vi "Create 3D Mecanum Wheel from Params.vi"(5 "colors":T2={"wheel color"=4884736, "roller color"=590024}, 7 "dimensions":T1={"roller thickness"=0.1, "roller radius"=0.05, "frame thickness"=0.025, "number of rollers"=6, "axle radius"=0.03, "axle length"=0.5}, 8 "error in (no error)":errorcluster, 9 "roller orientation":T3 items=["Left", "Right"], 10 "wheel radius":dbl=0.25, 11 "name":string) -> (0 "error out":errorcluster, 2 "rotation axis":refnum<vi>, 3 "3D mecanum wheel frame":refnum<vi>)   [LabVIEW 2017, in "NI_Robotics 3D Picture Steering Utilities.lvlib"]
doc: "Creates a 3D picture control mecanum wheel object."
uses:
  <vilib>/robotics/Steering/Utilities/3D Picture/NI_Robotics 3D Picture Steering Utilities.lvlib
  <vilib>/robotics/Steering/Mecanum Wheel/Roller Orientation.ctl
  <vilib>/robotics/Steering/Utilities/3D Picture/Mecanum Wheel Colors.ctl
  <vilib>/robotics/Steering/Utilities/3D Picture/Mecanum Wheel Dimensions.ctl
  <vilib>/picture/3D Picture Control/Object/Create Object (name).vi
  <vilib>/picture/3D Picture Control/NI_3D Picture Control.lvlib
  <vilib>/robotics/Steering/Mecanum Wheel/NI_Robotics_Mecanum Wheel.lvclass
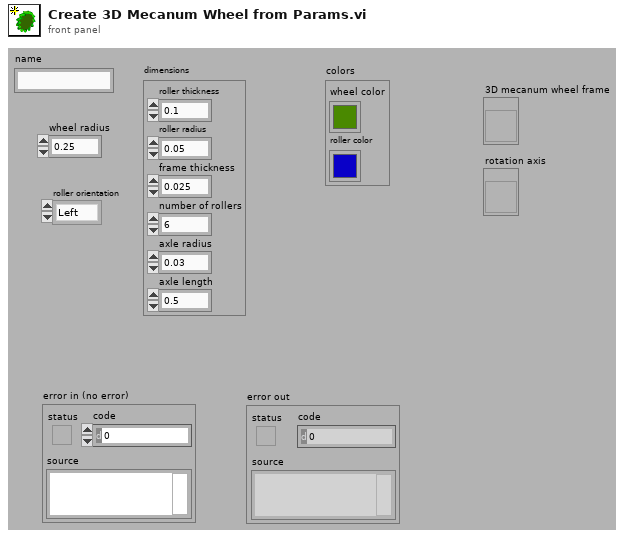
[diagram p1: front panel]
types:
  T1 = typedef "NI_Robotics 3D Picture Steering Utilities.lvlib/Mecanum Wheel Dimensions.ctl" = cluster{"roller thickness":dbl, "roller radius":dbl, "frame thickness":dbl, "number of rollers":i32, "axle radius":dbl, "axle length":dbl}
  T2 = typedef "NI_Robotics 3D Picture Steering Utilities.lvlib/Mecanum Wheel Colors.ctl" = cluster{"wheel color":u32, "roller color":u32}
  T3 = typedef "NI_Robotics_Mecanum Wheel.lvclass/Roller Orientation.ctl" = u16
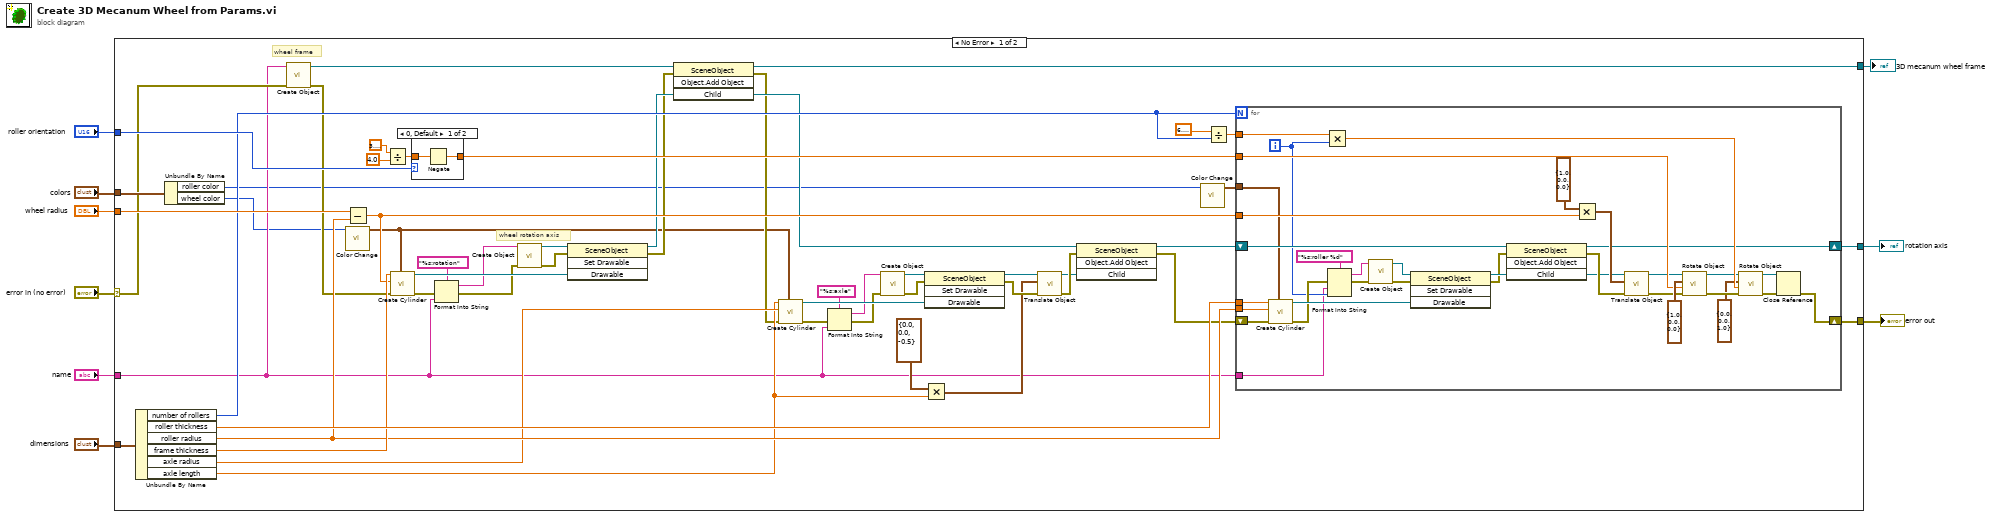
[diagram p0: block diagram]
diagram:
  n1 = case shown="No Error" "error in (no error)" {
    selector: "error in (no error)" -> [w26 w101]
    tunnel: [w59 _] -> w9
    tunnel: "dimensions" -> [w58 _]
    tunnel: "wheel radius" -> [w51 _]
    tunnel: "colors" -> [w49 _]
    tunnel: "roller orientation" -> [w28 _]
    tunnel: [w33 w101] -> w3
    tunnel: "name" -> [w15 _]
    tunnel: [w19 _] -> w1
    frame No Error {
      # "wheel rotation axis"
      # "wheel frame"
      n2 = Unbundle By Name(w58) -> ("number of rollers"=w27:i32, "roller thickness"=w57:dbl, "roller radius"=w52:dbl, "frame thickness"=w53:dbl, "axle radius"=w46:dbl, "axle length"=w36:dbl)
      n3 = Unbundle By Name(w49) -> ("roller color"=w11:u32, "wheel color"=w13:u32)
      n4 = call-poly <vilib>:"Create Object.vi"("error in (no error)"=w26, "Name"=w15) -> ("error out"=w25:errorcluster, "Scene:New Object"=w24:refnum<vi>)  [unwired: 8 in]
      n5 = call <vilib>:"Color Change.vi"("Color"=w13) -> ("RGBA"=w12:cluster{"R":sgl, "G":sgl, "B":sgl, "A":sgl})  [unwired: 10 in]
      n6 = Subtract(x=w51, y=w52) -> (x-y=w50:dbl)
      n7 = Divide(x=3.141592653589793, y=4.0) -> (x/y=w48:dbl)
      n8 = call <vilib>:"Create Cylinder.vi"("Color"=w12, "error in (no error)"=w25, "Radius"=w50, "Height"=w53) -> ("error out"=w18:errorcluster, "New Cylinder Refnum"=w56:refnum<vi>)  [unwired: 6 out]
      n9 = case shown="0, Default" w28 {
        tunnel: w48 -> [w65 w66]
        tunnel: [w64 w66] -> w47
        frame 0, Default {
          n10 = Negate(x=w65) -> (-x=w64:dbl)
        }
        frame 1 {
        }
      }
      n11 = Format Into String(format string="%s:rotation", error in=w18, w15) -> (resulting string=w14:string, error out=w17:errorcluster)  [unwired: 1 in]
      n12 = call-poly <vilib>:"Create Object.vi"("error in (no error)"=w17, "Name"=w14) -> ("error out"=w54:errorcluster, "Scene:New Object"=w55:refnum<vi>)  [unwired: 8 in]
      n13 = invoke class="SceneObject" method="Set Drawable"(reference=w55, error in=w54, "Drawable"=w56) -> (reference out=w23:refnum<vi>, error out=w21:errorcluster)  [unwired: 1 in, 2 out]
      n14 = invoke class="SceneObject" method="Object.Add Object"(reference=w24, error in=w21, "Child"=w23) -> (reference out=w19:refnum<vi>, error out=w20:errorcluster, "Child"=w22:refnum<vi>)  [unwired: 1 in, 1 out]
      n15 = call <vilib>:"Create Cylinder.vi"("Color"=w12, "error in (no error)"=w20, "Radius"=w46, "Height"=w36) -> ("error out"=w32:errorcluster, "New Cylinder Refnum"=w43:refnum<vi>)  [unwired: 6 out]
      n16 = Format Into String(format string="%s:axle" ("Name"), error in=w32, w15) -> (resulting string=w29:string, error out=w31:errorcluster)  [unwired: 1 in]
      n17 = call-poly <vilib>:"Create Object.vi"("error in (no error)"=w31, "Name"=w29) -> ("error out"=w44:errorcluster, "Scene:New Object"=w45:refnum<vi>)  [unwired: 8 in]
      n18 = invoke class="SceneObject" method="Set Drawable"(reference=w45, error in=w44, "Drawable"=w43) -> (reference out=w38:refnum<vi>, error out=w40:errorcluster)  [unwired: 1 in, 2 out]
      n19 = Multiply(x=cluster{"X":sgl, "Y":sgl, "Z":sgl} {"X"=0.0, "Y"=0.0, "Z"=-0.5} ("Translation"), y=w36) -> (x*y=w34:cluster{"X":dbl, "Y":dbl, "Z":dbl})
      n20 = call <vilib>:"Translate Object.vi"("error in (no error)"=w40, "Translation"=w34, "Scene.Object In"=w38) -> ("error out"=w39:errorcluster, "Scene.Object Out"=w37:refnum<vi>)  [unwired: 7 out]
      n21 = invoke class="SceneObject" method="Object.Add Object"(reference=w22, error in=w39, "Child"=w37) -> (reference out=w42:refnum<vi>, error out=w41:errorcluster)  [unwired: 1 in, 2 out]
      n22 = call <vilib>:"Color Change.vi"("Color"=w11) -> ("RGBA"=w10:cluster{"R":sgl, "G":sgl, "B":sgl, "A":sgl})  [unwired: 10 in]
      n23 = Divide(x=6.283185307179586, y=w27) -> (x/y=w62:dbl)
      n24 = for {
        N: w27 -> [_]
        tunnel: w52 -> [w100]
        tunnel: w50 -> [w89]
        tunnel: w62 -> [w93]
        shift-right: [w72] -> w33
        shift-left: w41 -> [w87]
        tunnel: w47 -> [w91]
        shift-right: [w71] -> w59
        shift-left: w42 -> [w74]
        tunnel: w57 -> [w70]
        tunnel: w10 -> [w69]
        tunnel: w15 -> [w67]
        i -> [w68]
        n25 = call <vilib>:"Create Cylinder.vi"("Color"=w69, "error in (no error)"=w87, "Radius"=w100, "Height"=w70) -> ("error out"=w86:errorcluster, "New Cylinder Refnum"=w95:refnum<vi>)  [unwired: 6 out]
        n26 = Multiply(x=w93, y=w68) -> (x*y=w92:dbl)
        n27 = Format Into String(format string="%s:roller %d", error in=w86, w67, w68) -> (resulting string=w75:string, error out=w98:errorcluster)  [unwired: 1 in]
        n28 = call-poly <vilib>:"Create Object.vi"("error in (no error)"=w98, "Name"=w75) -> ("error out"=w97:errorcluster, "Scene:New Object"=w96:refnum<vi>)  [unwired: 8 in]
        n29 = invoke class="SceneObject" method="Set Drawable"(reference=w96, error in=w97, "Drawable"=w95) -> (reference out=w85:refnum<vi>, error out=w73:errorcluster)  [unwired: 1 in, 2 out]
        n30 = invoke class="SceneObject" method="Object.Add Object"(reference=w74, error in=w73, "Child"=w85) -> (reference out=w71:refnum<vi>, error out=w84:errorcluster, "Child"=w83:refnum<vi>)  [unwired: 1 in, 1 out]
        n31 = Multiply(x=cluster{"X":sgl, "Y":sgl, "Z":sgl} {"X"=1.0, "Y"=0.0, "Z"=0.0} ("Translation"), y=w89) -> (x*y=w88:cluster{"X":dbl, "Y":dbl, "Z":dbl})
        n32 = call <vilib>:"Translate Object.vi"("error in (no error)"=w84, "Translation"=w88, "Scene.Object In"=w83) -> ("error out"=w82:errorcluster, "Scene.Object Out"=w81:refnum<vi>)  [unwired: 7 out]
        n33 = call <vilib>:"Rotate Object.vi"("error in (no error)"=w82, "Angle"=w91, "Axis"=cluster{"X":sgl, "Y":sgl, "Z":sgl} {"X"=1.0, "Y"=0.0, "Z"=0.0}, "Scene.Object In"=w81) -> ("error out"=w80:errorcluster, "Scene.Object Out"=w79:refnum<vi>)  [unwired: 6 out]
        n34 = call <vilib>:"Rotate Object.vi"("error in (no error)"=w80, "Angle"=w92, "Axis"=cluster{"X":sgl, "Y":sgl, "Z":sgl} {"X"=0.0, "Y"=0.0, "Z"=1.0}, "Scene.Object In"=w79) -> ("error out"=w77:errorcluster, "Scene.Object Out"=w78:refnum<vi>)  [unwired: 6 out]
        n35 = Close Reference(reference=w78, error in (no error)=w77) -> (error out=w72:errorcluster)
      }
    }
    frame Error {
    }
  }
  "rotation axis" <- w9
  "error out" <- w3
  "3D mecanum wheel frame" <- w1
